vi "Facade.vi"(0 "Data In":T6={"t0"=timestamp(0 s since 1904-01-01), "dt"=0.0, "Y"=[]}, 2 "Display State In":T4, 3 "Container State":T5) -> (6 "Data Out":T6, 7 "Display State Out":T4, 8 "Action":T3)   [LabVIEW 2018, in "Waveform Control.xctl"]
uses:
  Waveform Control.xctl
  Controls/Data.ctl
  <vilib>/_xctls/Container State.ctl
  Controls/State.ctl
  <vilib>/_xctls/Action.ctl
  subvis/FP Controls.ctl
  subvis/Function Types.ctl
  Controls/Volatile State Ops.ctl
  <vilib>/_xctls/XControlSupport.lvlib
panel:
  in  "Controls":T1={"Type"=enum."Sine", "Periods"=0.0, "Points"=2, "Offset"=0.0, "Amplitdue"=0.0, "Phase"=0.0, "func"=""} {"Points" min=1 step=1}
  out "Display":waveform(dbl)[](graph)
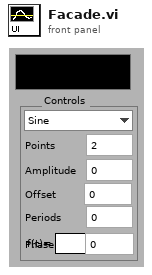
[diagram p1: front panel]
types:
  T1 = typedef "Waveform Control.xctl/FP Controls.ctl" = cluster{"Type":T2, "Periods":dbl, "Points":i32, "Offset":dbl, "Amplitdue":dbl, "Phase":dbl, "func":string}
  T2 = typedef "Waveform Control.xctl/Function Types.ctl" = enum16{"Level", "Sine", "Triangle", "Ramp", "Saw Tooth", "Square", "Function"}
  T3 = typedef "XControlSupport.lvlib/Action.ctl" = cluster{"Data Changed?":bool, "State Changed?":bool, "Action Name":string}
  T4 = typedef "Waveform Control.xctl/State.ctl" = cluster{"Name":string}
  T5 = typedef "XControlSupport.lvlib/Container State.ctl" = cluster{"Indicator?":bool, "Run Mode?":bool, " Refnum":refnum<vi>}
  T6 = typedef "Waveform Control.xctl/Data.ctl" = waveform(dbl)
  T7 = cluster{"Phase":refnum<vi>, "Amplitdue":refnum<vi>, "Points":refnum<vi>, "Type":refnum<vi>, "Periods":refnum<vi>, "func":refnum<vi>, "Offset":refnum<vi>}
  T8 = typedef "Waveform Control.xctl/Volatile State Ops.ctl" = enum16{"Read", "Write", "Update State from Data"}
  T9 = typedef "Waveform Control.xctl/Waveform State.ctl" = cluster{"Show Axes":bool, "Show Y=0":bool, "Controls":T1, "Show Current Location":bool, "Current Location":i32, "dt":dbl, "t0":timestamp, "Format and Units":string}
  T10 = typedef "LVRectTypeDef.ctl" = cluster{"Left":i16, "Top":i16, "Right":i16, "Bottom":i16}
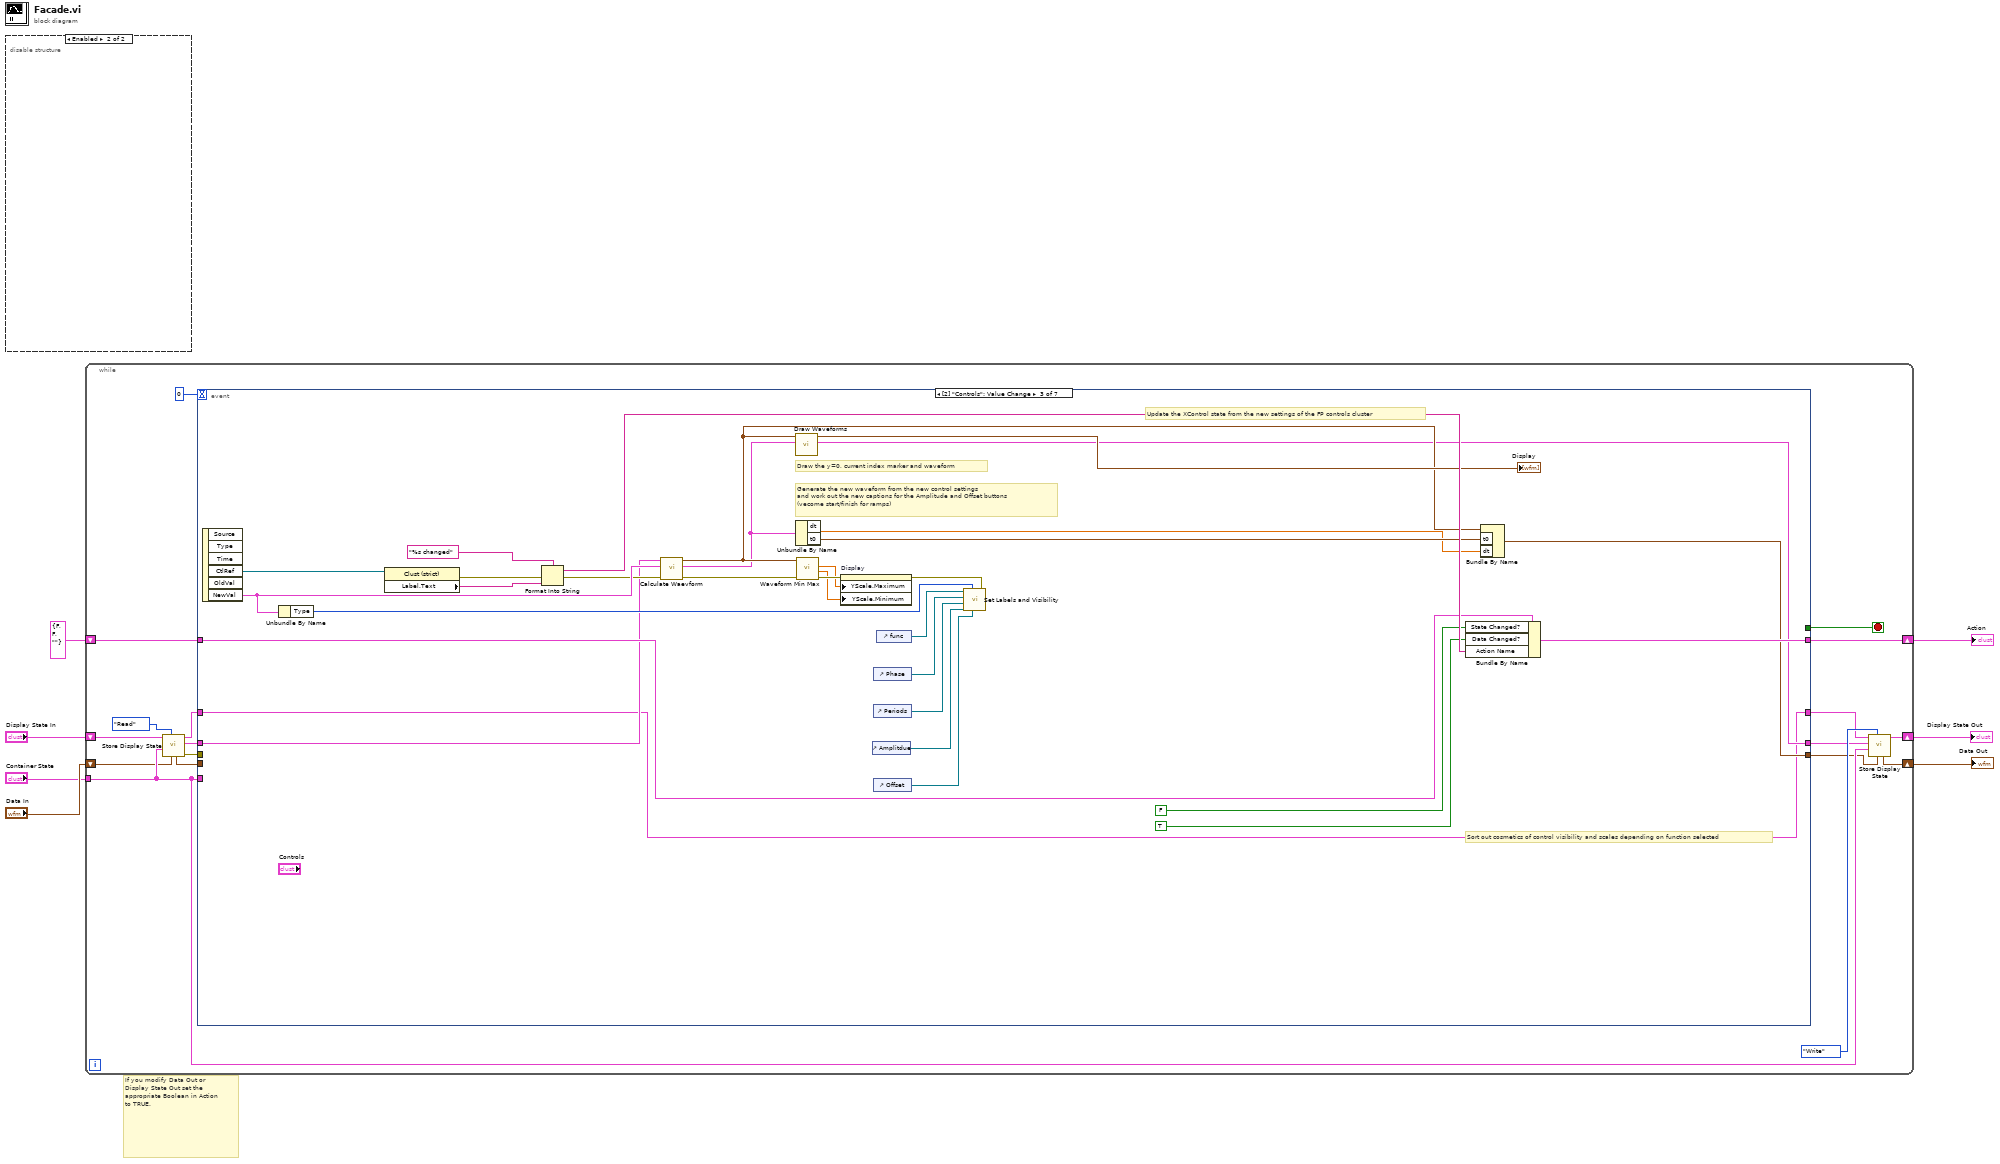
[diagram p0: block diagram]
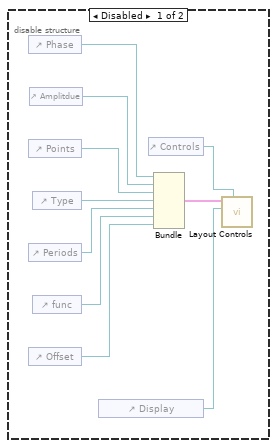
[diagram p2: hidden frame]
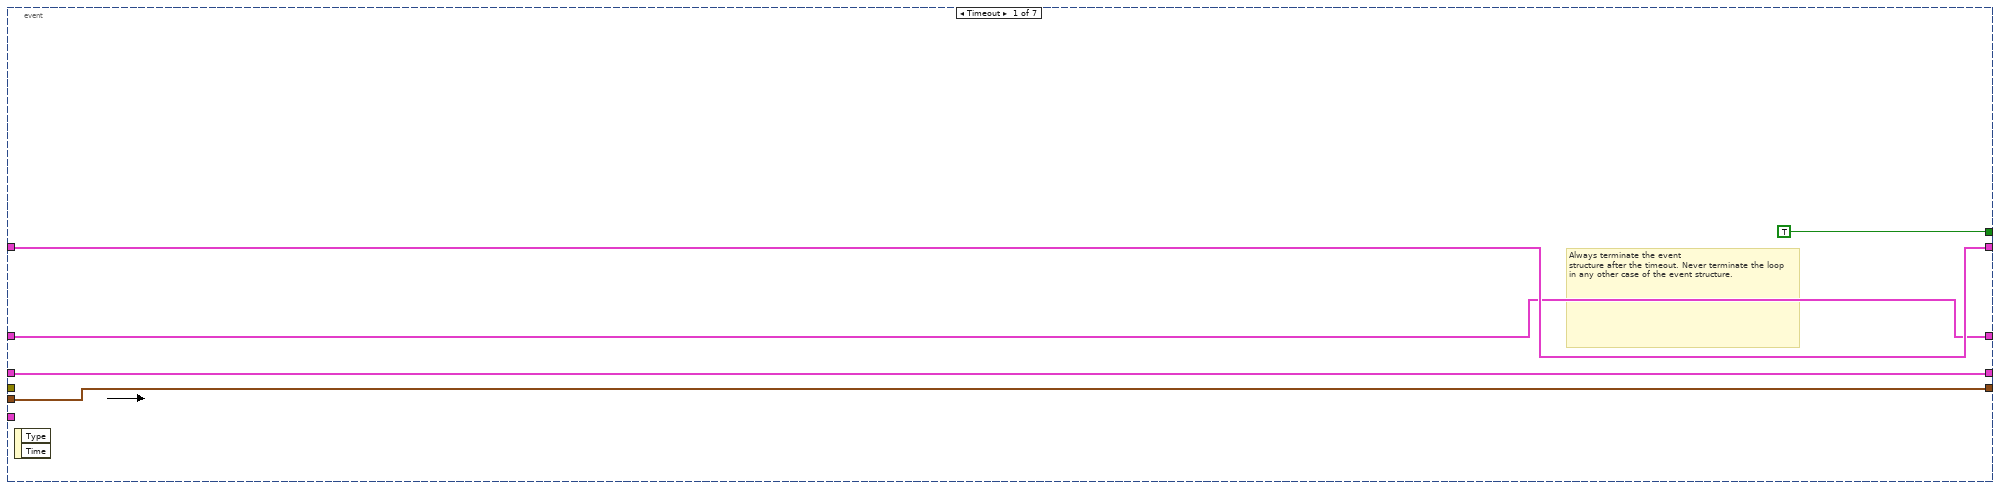
[diagram p3: hidden frame]
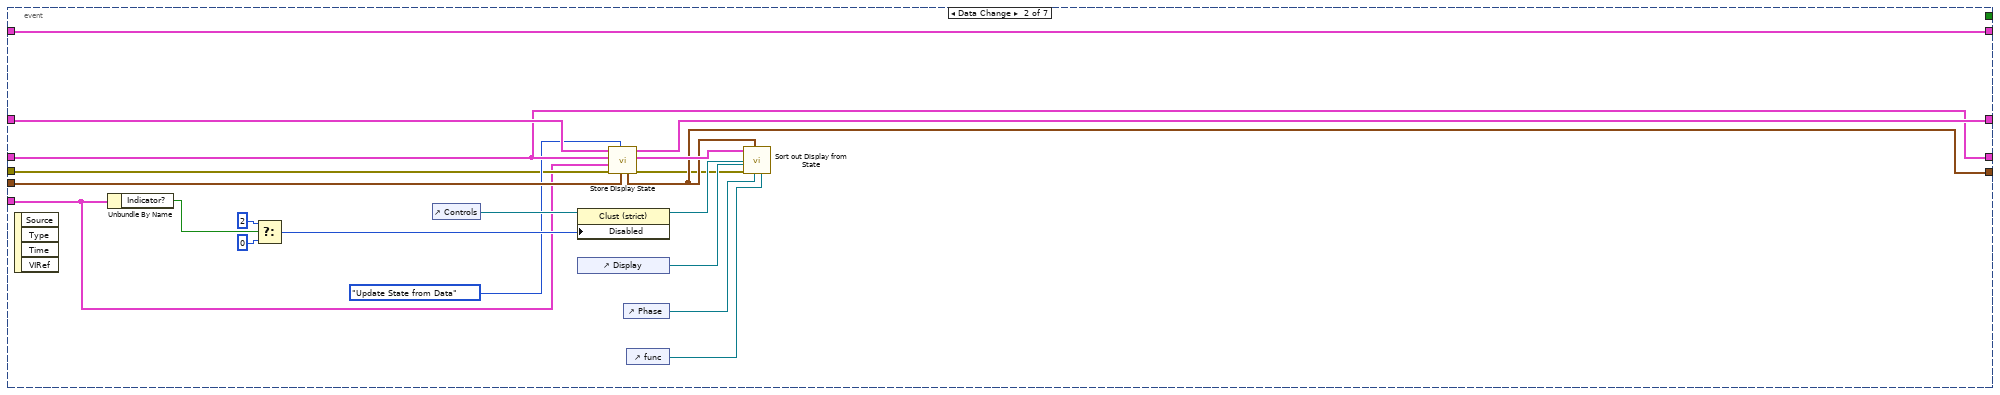
[diagram p4: hidden frame]
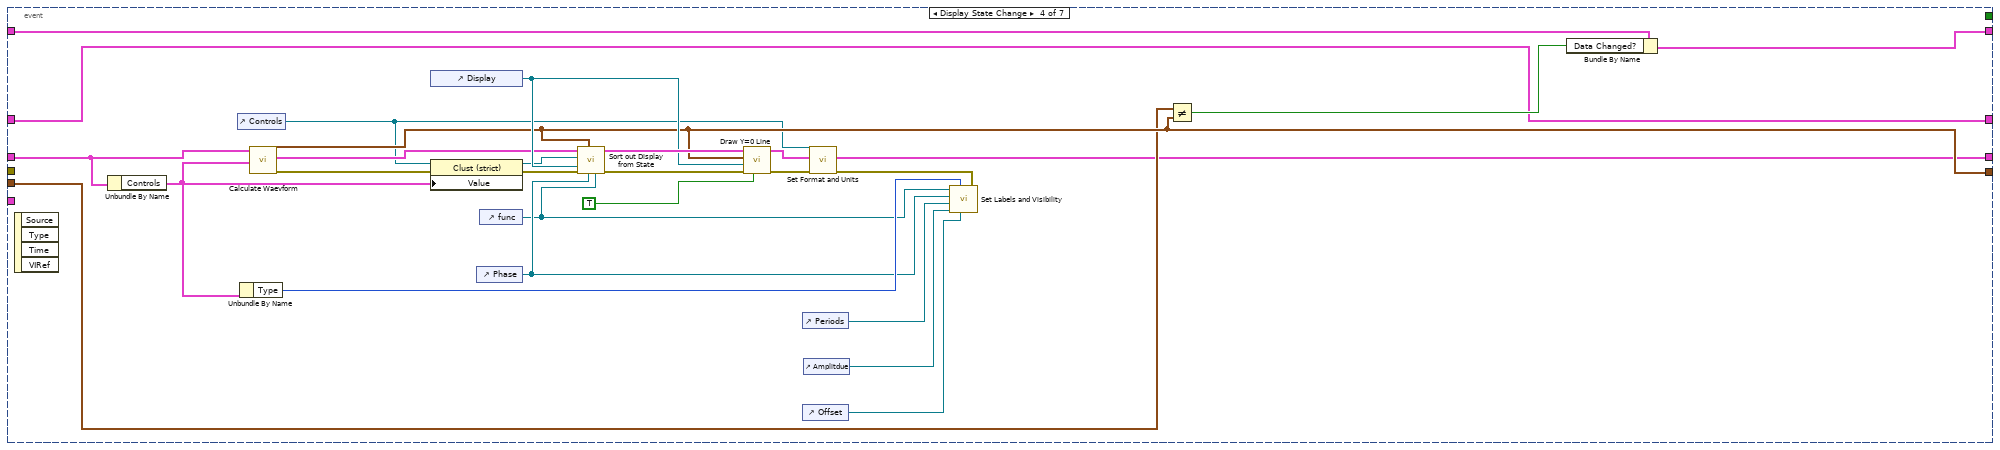
[diagram p5: hidden frame]
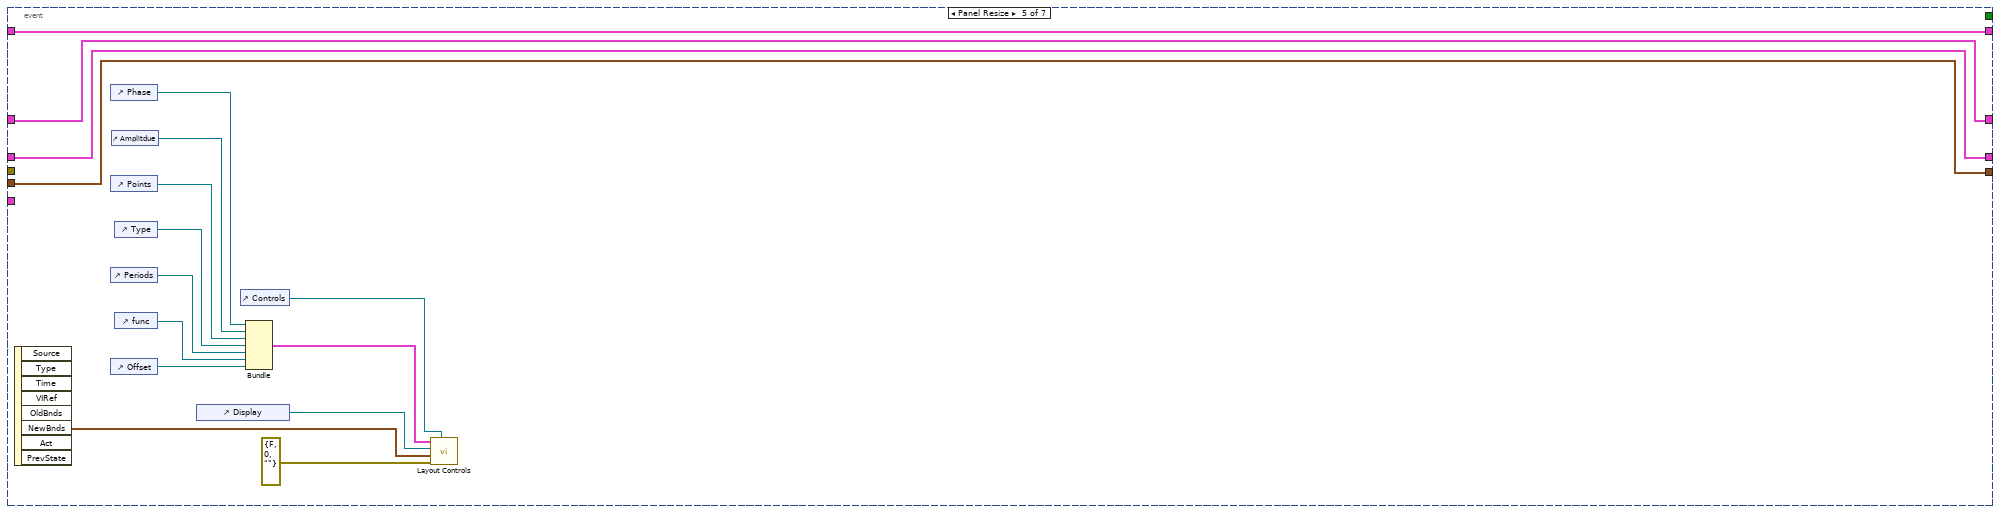
[diagram p6: hidden frame]
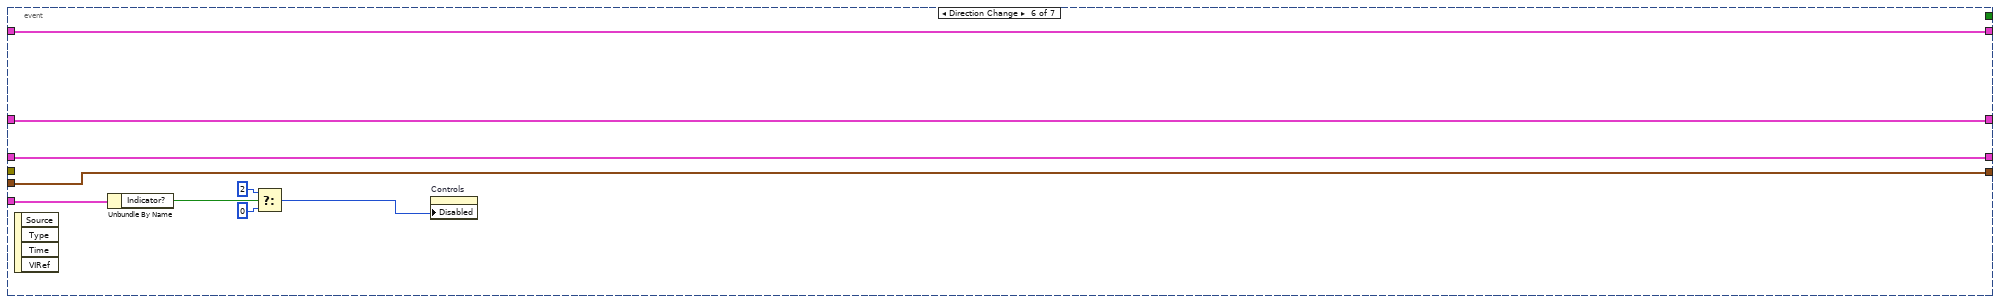
[diagram p7: hidden frame]
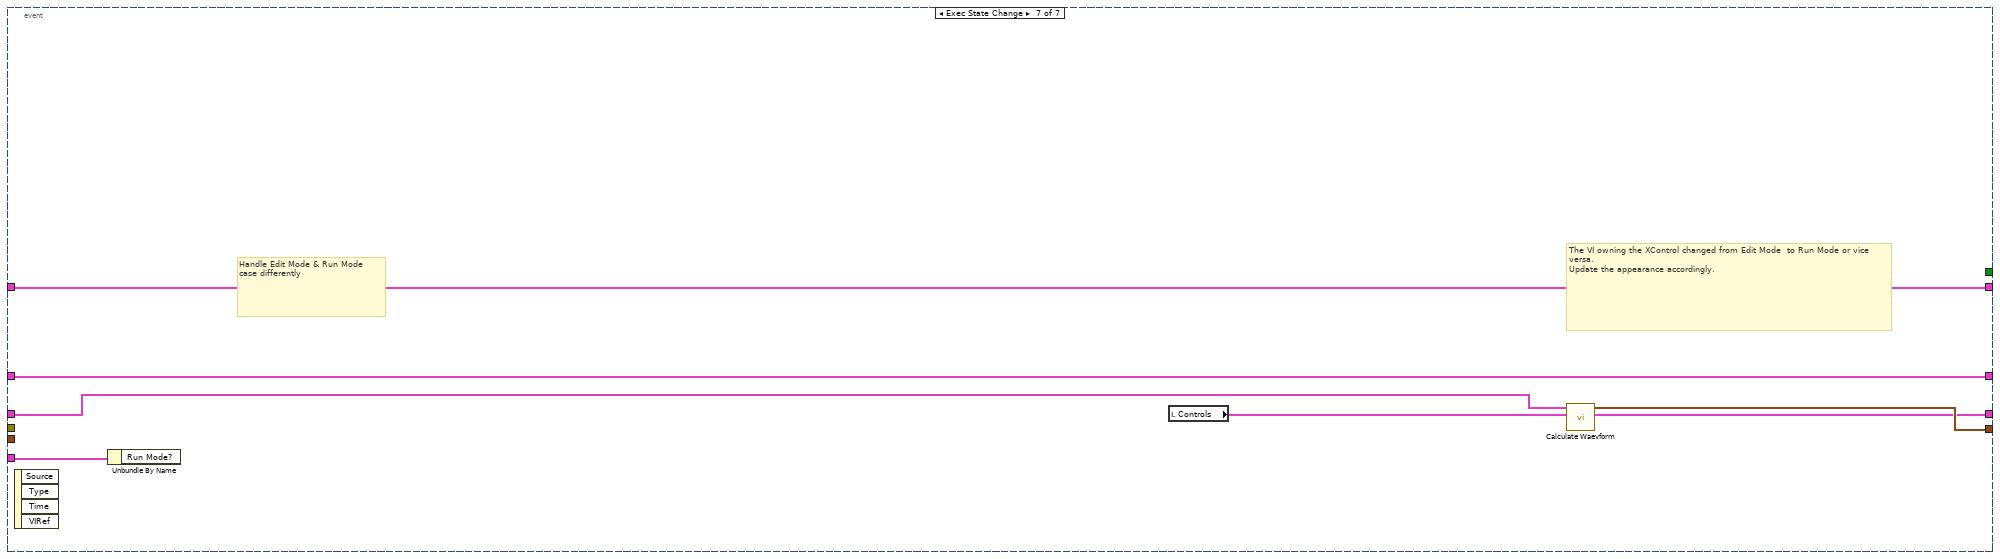
[diagram p8: hidden frame]
diagram:
  # "If you modify Data Out or\nDisplay State Out set the\nappropriate Boolean in Action\nto TRUE."
  n1 = disable-structure shown="Enabled" {
    frame Disabled {
      n2 = control-ref of="Phase"() -> (w8:refnum<vi>)
      n3 = control-ref of="Points"() -> (w10:refnum<vi>)
      n4 = control-ref of="Periods"() -> (w12:refnum<vi>)
      n5 = control-ref of="Offset"() -> (w14:refnum<vi>)
      n6 = control-ref of="Amplitdue"() -> (w9:refnum<vi>)
      n7 = control-ref of="Type"() -> (w11:refnum<vi>)
      n8 = control-ref of="func"() -> (w13:refnum<vi>)
      n9 = control-ref of="Display"() -> (w15:refnum<vi>)
      n10 = control-ref of="Controls"() -> (w17:refnum<vi>)
      n11 = Bundle("Phase"=w8, "Amplitdue"=w9, "Points"=w10, "Type"=w11, "Periods"=w12, "func"=w13, "Offset"=w14) -> (w16:T7)  [unwired: 1 out]
      n12 = call "Layout Controls.vi"("Control Cliuster In"=w17, "Waveform Ref In"=w15, "Controls Refs In"=w16) -> ()  [unwired: 6 in, 3 out]
    }
    frame Enabled {
    }
  }
  n13 = while {
    shift-right: [w30] -> w4
    shift-left: "Display State In" -> [w35]
    tunnel: "Container State" -> [w25]
    shift-right: [w21] -> w7
    shift-left: "Data In" -> [w24]
    shift-right: [w31] -> w2
    shift-left: T3 {"Data Changed?"=FALSE, "State Changed?"=FALSE, "Action Name"=""} ("Action") -> [w32]
    stop <- w34 stop-if-true
    n14 = call "Store Display State.vi"("Data In"=w24, "Operation In"=Volatile_State_Ops."Read", "Container State In"=w25, "State In"=w35) -> ("Error Out"=w18:errorcluster, "Waveform State Out"=w28:T9, "Display State Out"=w20:T4, "Data Out"=w23:T6)  [unwired: 2 in, 2 out]
    n15 = event shown="[2] \"Controls\": Value Change" {
      selector: _ -> [_ _ _ _ _ _ _]
      dyn-events: _ -> [_ _ _ _ _ _ _]
      timeout: 0 -> [_ _ _ _ _ _ _]
      tunnel: w28 -> [w38 w48 w67 w112 w133 w142 w145]
      tunnel: [w38 w48 w68 w101 w133 w142 w146] -> w27
      tunnel: [TRUE _ _ _ _ _ _] -> w34
      tunnel: w25 -> [_ w41 _ _ _ w143 w150]
      tunnel: w23 -> [w37 w50 _ w107 w134 w141 _]
      tunnel: [w37 w46 w75 w108 w134 w141 w147] -> w22
      tunnel: [w39 w42 w79 w117 w132 w140 w149] -> w31
      tunnel: w32 -> [w39 w42 w80 w118 w132 w140 w149]
      tunnel: w20 -> [w36 w51 w66 w105 w119 w135 w144]
      tunnel: [w36 w49 w66 w105 w119 w135 w144] -> w19
      tunnel: w18 -> [_ w43 _ _ _ _ _]
      event Timeout {
        # "Always terminate the event\nstructure after the timeout. Never terminate the loop in any other case of the event structure."
        n16 = event-data() -> ()  [unwired: 3 out]
      }
      event Data Change {
        n17 = event-data() -> ()  [unwired: 5 out]
        n18 = Unbundle By Name(w41) -> ("Indicator?"=w53:bool)
        n19 = Select(t=2, s=w53, f=0) -> (s? t:f=w56:i32)
        n20 = control-ref of="Controls"() -> (w60:refnum<vi>)
        n21 = property class="Clust (strict)"(reference=w60, "Disabled"=w56) -> (reference out=w52:refnum<vi>)  [unwired: 1 in, 1 out]
        n22 = control-ref of="Display"() -> (w57:refnum<vi>)
        n23 = call "Store Display State.vi"("Data In"=w50, "Operation In"=Volatile_State_Ops."Update State from Data", "Error In (no Error) In"=w43, "Container State In"=w41, "Waveform State In"=w48, "State In"=w51) -> ("Error Out"=w44:errorcluster, "Waveform State Out"=w47:T9, "Display State Out"=w49:T4, "Data Out"=w46:T6)  [unwired: 2 out]
        n24 = control-ref of="Phase"() -> (w58:refnum<vi>)
        n25 = control-ref of="func"() -> (w59:refnum<vi>)
        n26 = call "Sort out Display from State.vi"("Func In"=w59, "Starting Phase In"=w58, "Data In"=w46, "Error In (no Error) In"=w44, "Display In"=w57, "Controls In"=w52, "Display State In"=w47) -> ()  [unwired: 5 out]
      }
      event Value Change {
        # "Sort out cosmetics of control visibility and scales depending on function selected"
        # "Draw the y=0, current index marker and waveform"
        # "Generate the new waveform from the new control settings\nand work out the new captions for the Amplitude and Offset buttons\n(vecome start/finish for ramps)"
        # "Update the XControl state from the new settings of the FP controls cluster"
        n27 = event-data() -> ("CtlRef"=w91:refnum<vi>, "NewVal"=w73:T1)  [unwired: 5 out]
        n28 = Unbundle By Name(w73) -> ("Type"=w84:T2)
        n29 = property class="Clust (strict)"(reference=w91) -> (error out=w81:errorcluster, "Label.Text"=w89:string)  [unwired: 1 in, 1 out]
        n30 = Format Into String(format string="%s changed" ("Action Name"), error in=w81, w89) -> (resulting string=w88:string, error out=w71:errorcluster)  [unwired: 1 in]
        n31 = call "Calculate Waevform.vi"("Error In (no Error) In"=w71, "Controls In"=w73, "Display State In"=w67) -> ("Error Out"=w70:errorcluster, "Display State Out"=w69:T9, "Signal Out"=w72:waveform(dbl))  [unwired: 6 out]
        n32 = call "Draw Waveforms.vi"("Display State In"=w69, "Data In"=w72) -> ("Display State Out"=w68:T9, "Array Out"=→"Display":T6[])  [unwired: 1 in, 7 out]
        n33 = Unbundle By Name(w69) -> ("dt"=w77:dbl, "t0"=w78:timestamp)
        n34 = call <vilib>:"Waveform Min Max.vi"("error in (no error)"=w70, "waveform in"=w72) -> ("error out"=w87:errorcluster, "Y min"=w86:dbl, "Y max"=w85:dbl)  [unwired: 7 out]
        n35 = property on="Display" class="WFGraph (strict)"(error in=w87, "YScale.Maximum"=w85, "YScale.Minimum"=w86) -> (error out=w82:errorcluster)  [unwired: 1 in, 1 out]
        n36 = control-ref of="Amplitdue"() -> (w62:refnum<vi>)
        n37 = control-ref of="Phase"() -> (w64:refnum<vi>)
        n38 = control-ref of="Periods"() -> (w63:refnum<vi>)
        n39 = control-ref of="Offset"() -> (w61:refnum<vi>)
        n40 = control-ref of="func"() -> (w65:refnum<vi>)
        n41 = call "Set Labels and Visibility.vi"("error In"=w82, "Offset Refnum"=w61, "Type"=w84, "Amplitude Refnum"=w62, "Periods Renum"=w63, "Phase Refnum"=w64, "Function Refnum"=w65) -> ()  [unwired: 1 out]
        n42 = Bundle By Name(cluster=w80, "State Changed?"=FALSE, "Data Changed?"=TRUE ("State Changed?"), "Action Name"=w88) -> (w79:T3)
        n43 = Bundle By Name(cluster=w72, "t0"=w78, "dt"=w77) -> (w75:waveform(dbl))
      }
      event Display State Change {
        n44 = event-data() -> ()  [unwired: 5 out]
        n45 = Unbundle By Name(w112) -> ("Controls"=w95:T1)
        n46 = control-ref of="Controls"() -> (w100:refnum<vi>)
        n47 = Unbundle By Name(w95) -> ("Type"=w94:T2)
        n48 = call "Calculate Waevform.vi"("Controls In"=w95, "Display State In"=w112) -> ("Error Out"=w104:errorcluster, "Display State Out"=w111:T9, "Signal Out"=w108:waveform(dbl))  [unwired: 1 in, 6 out]
        n49 = control-ref of="Display"() -> (w114:refnum<vi>)
        n50 = property class="Clust (strict)"(reference=w100, error in=w104, "Value"=w95) -> (reference out=w109:refnum<vi>, error out=w110:errorcluster)
        n51 = control-ref of="Phase"() -> (w93:refnum<vi>)
        n52 = control-ref of="func"() -> (w92:refnum<vi>)
        n53 = call "Sort out Display from State.vi"("Func In"=w92, "Starting Phase In"=w93, "Data In"=w108, "Error In (no Error) In"=w110, "Display In"=w114, "Controls In"=w109, "Display State In"=w111) -> ("Error Out"=w116:errorcluster, "Display State Out"=w115:T9)  [unwired: 3 out]
        n54 = call "Draw Y=0 Line.vi"("Needs Update In"=TRUE ("Needs update"), "Error In (no Error) In"=w116, "PreviewGraph Ref In"=w114, "Data In"=w108, "Display State In"=w115) -> ("Error Ou Out"=w102:errorcluster, "Display State Out"=w103:T9)  [unwired: 2 in, 3 out]
        n55 = control-ref of="Periods"() -> (w99:refnum<vi>)
        n56 = control-ref of="Offset"() -> (w97:refnum<vi>)
        n57 = control-ref of="Amplitdue"() -> (w98:refnum<vi>)
        n58 = call "Set Format and Units.vi"("error in (no error)"=w102, "Display State In"=w103, "Cluster Control"=w100) -> ("error out"=w96:errorcluster, "Display State Out"=w101:T9)  [unwired: 7 out]
        n59 = call "Set Labels and Visibility.vi"("error In"=w96, "Offset Refnum"=w97, "Type"=w94, "Amplitude Refnum"=w98, "Periods Renum"=w99, "Phase Refnum"=w93, "Function Refnum"=w92) -> ()  [unwired: 1 out]
        n60 = Not Equal?(x=w107, y=w108) -> (x != y?=w106:bool)
        n61 = Bundle By Name(cluster=w118, "Data Changed?"=w106) -> (w117:T3)
      }
      event Panel Resize {
        n62 = event-data() -> ("NewBnds"=w122:T10)  [unwired: 8 out]
        n63 = control-ref of="Phase"() -> (w131:refnum<vi>)
        n64 = control-ref of="Points"() -> (w129:refnum<vi>)
        n65 = control-ref of="Periods"() -> (w127:refnum<vi>)
        n66 = control-ref of="Offset"() -> (w125:refnum<vi>)
        n67 = control-ref of="Amplitdue"() -> (w130:refnum<vi>)
        n68 = control-ref of="Type"() -> (w128:refnum<vi>)
        n69 = control-ref of="func"() -> (w126:refnum<vi>)
        n70 = control-ref of="Display"() -> (w123:refnum<vi>)
        n71 = control-ref of="Controls"() -> (w120:refnum<vi>)
        n72 = Bundle("Phase"=w131, "Amplitdue"=w130, "Points"=w129, "Type"=w128, "Periods"=w127, "func"=w126, "Offset"=w125) -> (w121:T7)  [unwired: 1 out]
        n73 = call "Layout Controls.vi"("Control Cliuster In"=w120, "Error In"=errorcluster {"status"=FALSE, "code"=0, "source"=""} ("error out"), "NewBnds In"=w122, "Waveform Ref In"=w123, "Controls Refs In"=w121) -> ()  [unwired: 4 in, 3 out]
      }
      event Direction Change {
        n74 = event-data() -> ()  [unwired: 5 out]
        n75 = Unbundle By Name(w143) -> ("Indicator?"=w139:bool)
        n76 = Select(t=2, s=w139, f=0) -> (s? t:f=w136:i32)
        n77 = property on="Controls" class="Clust (strict)"("Disabled"=w136) -> ()  [unwired: 2 in, 2 out]
      }
      event Exec State Change {
        # "The VI owning the XControl changed from Edit Mode  to Run Mode or vice versa.\nUpdate the appearance accordingly."
        # "Handle Edit Mode & Run Mode\ncase differently"
        n78 = event-data() -> ()  [unwired: 5 out]
        n79 = Unbundle By Name(w150) -> ()  [unwired: 1 out]
        n80 = local read "Controls"() -> (w148:T1)
        n81 = call "Calculate Waevform.vi"("Controls In"=w148, "Display State In"=w145) -> ("Display State Out"=w146:T9, "Signal Out"=w147:waveform(dbl))  [unwired: 1 in, 7 out]
      }
    }
    n82 = call "Store Display State.vi"("Data In"=w22, "Operation In"=Volatile_State_Ops."Write", "Container State In"=w25, "Waveform State In"=w27, "State In"=w19) -> ("Display State Out"=w30:T4, "Data Out"=w21:T6)  [unwired: 1 in, 4 out]
  }
  "Display State Out" <- w4
  "Data Out" <- w7
  "Action" <- w2
